vi "ma_Equi-RippleFIRCoeff.vi"(5 "sampling freq: fs":dbl=1.0 format="%0.2f", 6 "# of taps":i32=32, 7 "Filter type":T1(ring), 8 "higher stop freq":dbl=0.4000000000000001 format="%0.2f", 9 "higher pass freq":dbl=0.3500000000000001 format="%0.2f", 10 "lower stop freq":dbl=0.2 format="%0.2f", 11 "lower pass freq":dbl=0.25000000000000006 format="%0.2f") -> (0 "error":i32, 2 "ripple":dbl format="%0.2f", 3 "FIR Coefficients":dbl[](array[numeric]) format="%0.2f")   [LabVIEW 2020, in "NI_MAPro.lvlib"]
doc: "Bandpass filters the input sequence using the Equi-Ripple FIR filter model.\n\nFor more information, see the description of the following VI's:\n\n Parks-McClellan\n Convolution."
uses:
  NI_MAPro.lvlib
  NI_AALBase.lvlib
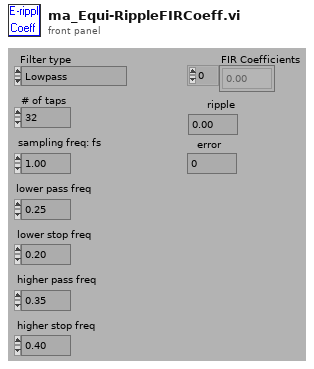
[diagram p1: front panel]
types:
  T1 = enum32{"Lowpass", "Highpass", "Bandpass", "Bandstop"}
  T2 = cluster{"Amplitude":dbl, "DC":dbl, "lower pass freq":dbl, "Weight":dbl}
  T3 = cluster{"Amplitude":dbl, "lower stop freq":dbl, dbl, "Weight":dbl}
  T4 = cluster{"Amplitude":dbl, "lower stop freq":dbl, "lower pass freq":dbl, "Weight":dbl}[]
  T5 = cluster{"Amplitude":dbl, "DC":dbl, "lower stop freq":dbl, "Weight":dbl}
  T6 = cluster{"Amplitude":dbl, "lower pass freq":dbl, dbl, "Weight":dbl}
  T7 = cluster{"Amplitude":dbl, "lower pass freq":dbl, "lower stop freq":dbl, "Weight":dbl}[]
  T8 = cluster{"Amplitude":dbl, "lower pass freq":dbl, "higher pass freq":dbl, "Weight":dbl}
  T9 = cluster{"Amplitude":dbl, "higher stop freq":dbl, dbl, "Weight":dbl}
  T10 = cluster{"Amplitude":dbl, "higher stop freq":dbl, "higher pass freq":dbl, "Weight":dbl}[]
  T11 = cluster{"Amplitude":dbl, "lower stop freq":dbl, "higher stop freq":dbl, "Weight":dbl}
  T12 = cluster{"Amplitude":dbl, "higher pass freq":dbl, dbl, "Weight":dbl}
  T13 = cluster{"Amplitude":dbl, "higher pass freq":dbl, "higher stop freq":dbl, "Weight":dbl}[]
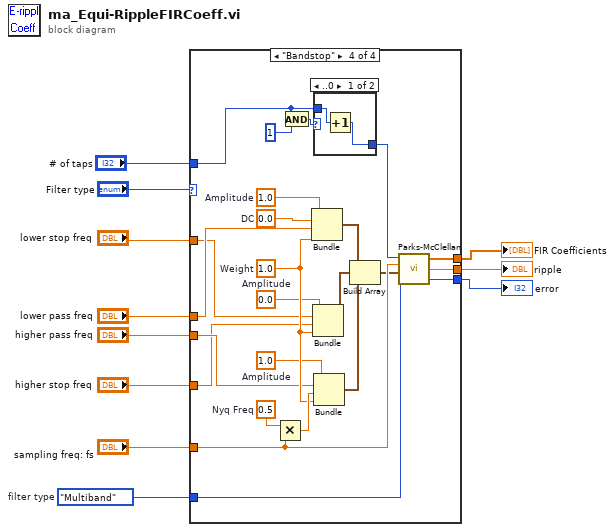
[diagram p0: block diagram]
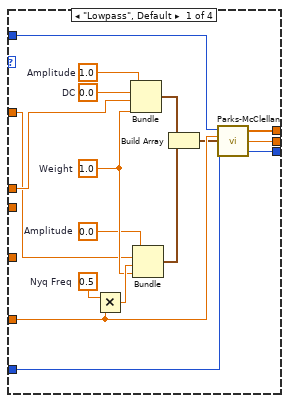
[diagram p2: hidden frame]
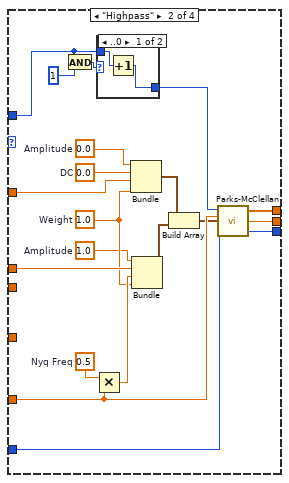
[diagram p3: hidden frame]
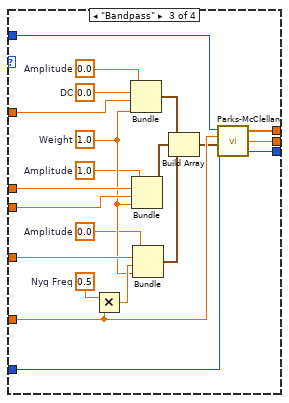
[diagram p5: hidden frame]
diagram:
  w6 = enum32{"Multiband", "Differentiator", "Hilbert"}."Multiband"  # filter type
  n1 = case shown="\"Bandstop\"" "Filter type" {
    tunnel: "lower stop freq" -> [w12 w33 w72 w75]
    tunnel: "lower pass freq" -> [w13 w48 w71 w76]
    tunnel: "higher pass freq" -> [_ _ w68 w74]
    tunnel: "higher stop freq" -> [_ _ w67 w73]
    tunnel: "sampling freq: fs" -> [w25 w44 w64 w92]
    tunnel: w6 -> [w23 w42 w62 w90]
    tunnel: [w18 w36 w55 w83] -> w5
    tunnel: [w17 w35 w54 w82] -> w4
    tunnel: [w16 w34 w53 w81] -> w3
    tunnel: "# of taps" -> [w15 w30 w52 w78]
    frame "Lowpass", Default {
      w19 = 0.5  # Nyq Freq
      w14 = 0.0  # Amplitude
      w20 = 1.0  # Weight
      w21 = 0.0  # DC
      w22 = 1.0  # Amplitude
      n2 = Multiply(x=w19, y=w25) -> (x*y=w27:dbl)
      n3 = Bundle("Amplitude"=w22, "DC"=w21, "lower pass freq"=w13, "Weight"=w20) -> (w28:T2)  [unwired: 1 in]
      n4 = Bundle("Amplitude"=w14, "lower stop freq"=w12, w27, "Weight"=w20) -> (w26:T3)  [unwired: 1 in]
      n5 = Build Array(w28, w26) -> (w24:T4)
      n6 = call "Parks-McClellan.vi"("filter type"=w23, "Band Parameters"=w24, "sampling freq: fs"=w25, "# of taps"=w15) -> ("error"=w18:i32, "ripple"=w16:dbl, "h"=w17:dbl[])
    }
    frame "Highpass" {
      w37 = 0.5  # Nyq Freq
      w38 = 1.0  # Amplitude
      w39 = 1.0  # Weight
      w40 = 0.0  # DC
      w41 = 0.0  # Amplitude
      n7 = And(x=w30, y=1) -> (x .and. y?=w31:i32)
      n8 = Multiply(x=w37, y=w44) -> (x*y=w45:dbl)
      n9 = case shown="..0" w31 {
        tunnel: w30 -> [w50 w51]
        tunnel: [w49 w51] -> w29
        frame ..0 {
          n10 = Increment(x=w50) -> (x+1=w49:i32)
        }
        frame 1.. {
        }
      }
      n11 = Bundle("Amplitude"=w41, "DC"=w40, "lower stop freq"=w33, "Weight"=w39) -> (w47:T5)  [unwired: 1 in]
      n12 = Bundle("Amplitude"=w38, "lower pass freq"=w48, w45, "Weight"=w39) -> (w46:T6)  [unwired: 1 in]
      n13 = Build Array(w47, w46) -> (w43:T7)
      n14 = call "Parks-McClellan.vi"("filter type"=w42, "Band Parameters"=w43, "sampling freq: fs"=w44, "# of taps"=w29) -> ("error"=w36:i32, "ripple"=w34:dbl, "h"=w35:dbl[])
    }
    frame "Bandpass" {
      w57 = 0.0  # Amplitude
      w56 = 0.5  # Nyq Freq
      w58 = 1.0  # Amplitude
      w59 = 1.0  # Weight
      w60 = 0.0  # DC
      w61 = 0.0  # Amplitude
      n15 = Multiply(x=w56, y=w64) -> (x*y=w66:dbl)
      n16 = Bundle("Amplitude"=w61, "DC"=w60, "lower stop freq"=w72, "Weight"=w59) -> (w70:T5)  [unwired: 1 in]
      n17 = Bundle("Amplitude"=w58, "lower pass freq"=w71, "higher pass freq"=w68, "Weight"=w59) -> (w69:T8)  [unwired: 1 in]
      n18 = Bundle("Amplitude"=w57, "higher stop freq"=w67, w66, "Weight"=w59) -> (w65:T9)  [unwired: 1 in]
      n19 = Build Array(w70, w69, w65) -> (w63:T10)
      n20 = call "Parks-McClellan.vi"("filter type"=w62, "Band Parameters"=w63, "sampling freq: fs"=w64, "# of taps"=w52) -> ("error"=w55:i32, "ripple"=w53:dbl, "h"=w54:dbl[])
    }
    frame "Bandstop" {
      w85 = 1.0  # Amplitude
      w84 = 0.5  # Nyq Freq
      w86 = 0.0  # Amplitude
      w87 = 1.0  # Weight
      w88 = 0.0  # DC
      w89 = 1.0  # Amplitude
      n21 = Multiply(x=w84, y=w92) -> (x*y=w94:dbl)
      n22 = And(x=w78, y=1) -> (x .and. y?=w79:i32)
      n23 = Bundle("Amplitude"=w89, "DC"=w88, "lower pass freq"=w76, "Weight"=w87) -> (w96:T2)  [unwired: 1 in]
      n24 = Bundle("Amplitude"=w86, "lower stop freq"=w75, "higher stop freq"=w73, "Weight"=w87) -> (w95:T11)  [unwired: 1 in]
      n25 = case shown="..0" w79 {
        tunnel: w78 -> [w98 w99]
        tunnel: [w97 w99] -> w77
        frame ..0 {
          n26 = Increment(x=w98) -> (x+1=w97:i32)
        }
        frame 1.. {
        }
      }
      n27 = Bundle("Amplitude"=w85, "higher pass freq"=w74, w94, "Weight"=w87) -> (w93:T12)  [unwired: 1 in]
      n28 = Build Array(w96, w95, w93) -> (w91:T13)
      n29 = call "Parks-McClellan.vi"("filter type"=w90, "Band Parameters"=w91, "sampling freq: fs"=w92, "# of taps"=w77) -> ("error"=w83:i32, "ripple"=w81:dbl, "h"=w82:dbl[])
    }
  }
  "FIR Coefficients" <- w4
  "error" <- w5
  "ripple" <- w3
